vi "Ammeter Configure (648X).vi"(8 "error in (no error)":errorcluster, 11 "VISA resource name in":refnum<visa-resource-name>) -> (0 "error out":errorcluster, 3 "VISA resource name out":refnum<visa-resource-name>)   [LabVIEW 2016, in "Hall Effect Library.lvlib"]
uses:
  Hall Effect Library.lvlib
  Global Variables/Test Settings.vi
  <instrlib>/Keithley 648X/Keithley 648X.lvlib
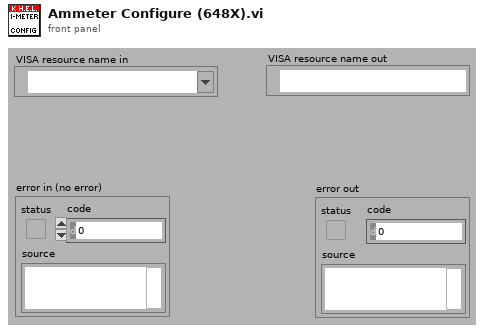
[diagram p1: front panel]
types:
  T1 = enum16{"2 nA", "20 nA", "200 nA", "2 uA", "20 uA", "200 uA", "2 mA", "20 mA"}
  T2 = enum16{"Auto", "2 nA", "20 nA", "200 nA", "2 uA", "20 uA", "200 uA", "2 mA", "20 mA"}
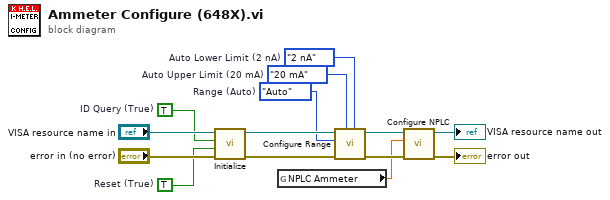
[diagram p0: block diagram]
diagram:
  w6 = TRUE  # Reset (True)
  w7 = TRUE  # ID Query (True)
  w10 = T1."2 nA"  # Auto Lower Limit (2 nA)
  w11 = T1."20 mA"  # Auto Upper Limit (20 mA)
  w12 = T2."Auto"  # Range (Auto)
  n1 = call <instrlib>:"Initialize.vi"("error in (no error)"="error in (no error)", "Reset (True)"=w6, "ID Query (True)"=w7, "VISA resource name"="VISA resource name in") -> ("error out"=w14:errorcluster, "VISA resource name out"=w13:refnum<visa-resource-name>)  [unwired: 1 in, 5 out]
  n2 = global read "Test Settings.vi" "NPLC Ammeter"() -> (w1:dbl)
  n3 = call <instrlib>:"Configure Range.vi"("Auto Lower Limit (2 nA)"=w10, "Auto Upper Limit (20 mA)"=w11, "error in"=w14, "Range (Auto)"=w12, "VISA resource name"=w13) -> ("error out"=w5:errorcluster, "VISA resource name out"=w4:refnum<visa-resource-name>)  [unwired: 5 out]
  n4 = call <instrlib>:"Configure NPLC.vi"("error in (no error)"=w5, "Powerline Cycles (1.000)"=w1, "VISA resource name"=w4) -> ("error out"=→"error out":errorcluster, "VISA resource name out"=→"VISA resource name out":refnum<visa-resource-name>)  [unwired: 7 out]
